vi "2.3.vi"() -> ()   [LabVIEW 2017]
panel:
  out "数值":dbl
  in  "b":dbl
  in  "x":dbl
  in  "k":dbl
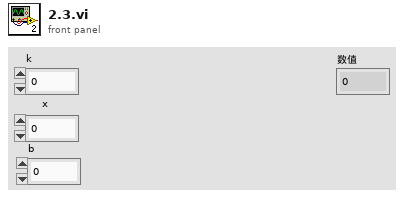
[diagram p1: front panel]
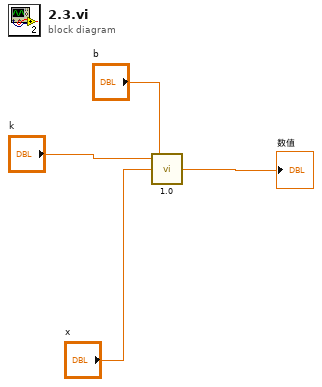
[diagram p0: block diagram]
diagram:
  n1 = call "1.0.vi"("b"="b", "x"="x", "k"="k") -> ("数值"=→"数值":dbl)
